vi "PiezoLaserMove010.vi"(8 "error in (no error)":errorcluster, 10 "Y":dbl, 11 "X":dbl) -> (0 "error out":errorcluster)   [LabVIEW 2011]
uses:
  <vilib>/DAQmx/create/channels.llb/DAQmx Create Channel (AO-Voltage-Basic).vi
  <vilib>/DAQmx/write.llb/DAQmx Write (Analog 1D DBL NChan 1Samp).vi
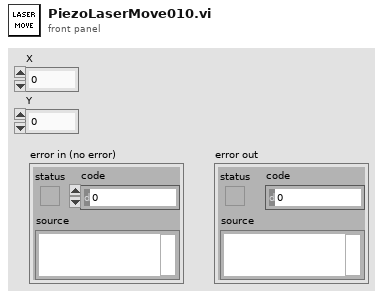
[diagram p1: front panel]
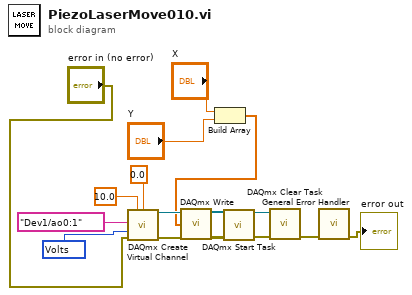
[diagram p0: block diagram]
diagram:
  w8 = 10348 items=["Volts"=10348, "From Custom Scale"=10065] ("units")
  n1 = call-poly <vilib>:"DAQmx Create Virtual Channel.vi"("maximum value"=10.0, "minimum value"=0.0, "physical channels"=tag "Dev1/ao0:1", "units"=w8, "error in"="error in (no error)") -> ("task out"=w14:refnum<k21>, "error out"=w15:errorcluster)  [unwired: 9 in]
  n2 = Build Array("X", "Y") -> (w3:dbl[])
  n3 = call-poly <vilib>:"DAQmx Write.vi"("task/channels in"=w14, "data"=w3, "error in"=w15) -> ("task out"=w11:refnum<k21>, "error out"=w13:errorcluster)  [unwired: 10 in, 1 out]
  n4 = call <vilib>:"DAQmx Start Task.vi"("task/channels in"=w11, "error in"=w13) -> ("task out"=w12:refnum<k21>, "error out"=w9:errorcluster)  [unwired: 12 in]
  n5 = call <vilib>:"DAQmx Clear Task.vi"("task in"=w12, "error in"=w9) -> ("error out"=w10:errorcluster)  [unwired: 13 in]
  n6 = call <vilib>:"General Error Handler.vi"("error in (no error)"=w10) -> ("error out"=→"error out":errorcluster)  [unwired: 10 in, 4 out]
